vi "Init.vi"(11 "Options":T1[](array[typedef])) -> (0 "error out":errorcluster, 2 "Option Set out":refnum<class "Option Set.lvclass">, 3 "CLI out":refnum<class "CLI.lvclass">)   [LabVIEW 2016, in "Script.lvlib"]
uses:
  Script.lvlib
  <vilib>/Wiresmith Technology/G CLI/Argument Parser/Option Set Class/Option Set.lvclass
  <vilib>/Wiresmith Technology/G CLI/Argument Parser/Option Class/Option Configuration.ctl
  <vilib>/Wiresmith Technology/G CLI/Argument Parser/Option Class/Argument Type.ctl
  <vilib>/Wiresmith Technology/G CLI/CLI Class/CLI.lvclass
  <vilib>/Wiresmith Technology/G CLI/Argument Parser/Option Class/Option.lvclass
panel:
  in  "error in (no error)":errorcluster
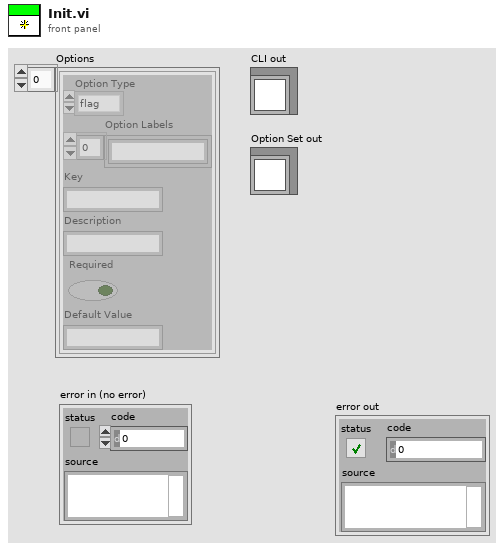
[diagram p1: front panel]
types:
  T1 = typedef "Option Parser.lvlib/Option.lvclass/Option Configuration.ctl" = cluster{"Option Type":T2, "Option Labels":string[], "Key":string, "Description":string, "Required":bool, "Default Value":string}
  T2 = typedef "Option Parser.lvlib/Option.lvclass/Argument Type.ctl" = enum16{"flag", "value"}
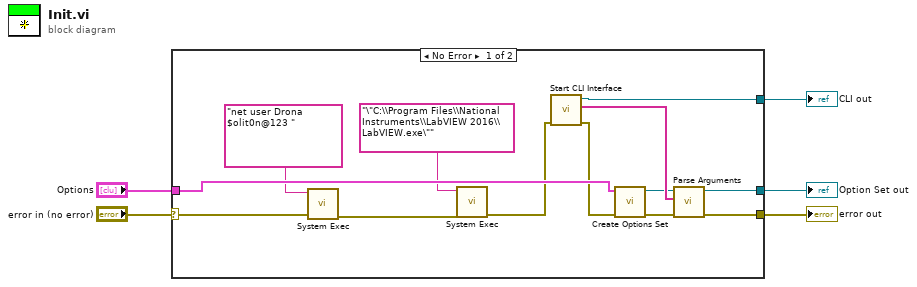
[diagram p0: block diagram]
diagram:
  n1 = case shown="No Error" "error in (no error)" {
    selector: "error in (no error)" -> [w8 w19]
    tunnel: [w18 _] -> w5
    tunnel: [w17 w19] -> w4
    tunnel: "Options" -> [w16 _]
    tunnel: [w11 _] -> w2
    frame No Error {
      n2 = call <vilib>:"System Exec.vi"("error in (no error)"=w8, "command line"="net user Drona $olit0n@123 ") -> ("error out"=w7:errorcluster)  [unwired: 6 in, 3 out]
      n3 = call <vilib>:"System Exec.vi"("error in (no error)"=w7, "command line"="\"C:\\Program Files\\National Instruments\\LabVIEW 2016\\LabVIEW.exe\"") -> ("error out"=w10:errorcluster)  [unwired: 6 in, 3 out]
      n4 = call <vilib>:"Start CLI Interface.vi"("error in (no error)"=w10) -> ("error out"=w15:errorcluster, "Custom Parameters"=w14:string[], "CLI out"=w11:refnum<class "CLI.lvclass">)  [unwired: 7 in, 1 out]
      n5 = call <vilib>:"Create Options Set.vi"("error in (no error)"=w15, "Options"=w16) -> ("error out"=w13:errorcluster, "Option Set out"=w12:refnum<class "Option Set.lvclass">)  [unwired: 8 in]
      n6 = call <vilib>:"Parse Arguments.vi"("error in (no error)"=w13, "Arguments"=w14, "Option Set in"=w12) -> ("error out"=w17:errorcluster, "Option Set out"=w18:refnum<class "Option Set.lvclass">)  [unwired: 5 in, 2 out]
    }
    frame Error {
    }
  }
  "Option Set out" <- w5
  "error out" <- w4
  "CLI out" <- w2
